vi "Apply (Greyscale Image).vi"(8 "error in (no error)":errorcluster, 9 "Destination Image in":T1, 10 "Greyscale Image in":T1, 11 "CLAHE in":refnum<class "CLAHE.lvclass">) -> (0 "error out":errorcluster, 2 "Destination Image":T1, 3 "CLAHE":refnum<class "CLAHE.lvclass">)   [LabVIEW 2020, in "image.lvlib" / "CLAHE.lvclass"]
uses:
  CLAHE.lvclass
  Greyscale Image.ctl
  CLAHE.lvclass/CLAHE.ctl
  common/common.lvlib
  common/bin/gartoolkit_32-1.dll
  image.lvlib
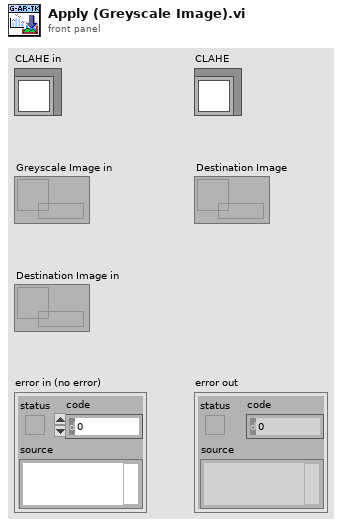
[diagram p1: front panel]
types:
  T1 = typedef "image.lvlib/Greyscale Image.ctl" = refnum<data-value>
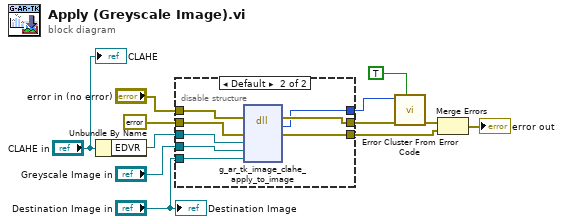
[diagram p0: block diagram]
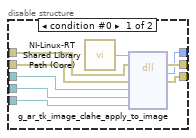
[diagram p2: hidden frame]
diagram:
  n1 = Unbundle By Name("CLAHE in") -> ("EDVR"=w1:refnum<data-value>)
  n2 = disable-structure shown="Default" {
    disable-tunnel: "error in (no error)" -> [w20 w29]
    disable-tunnel: errorcluster {"status"=FALSE, "code"=0, "source"=""} ("error constant") -> [w18 w28]
    disable-tunnel: w1 -> [w17 w24]
    disable-tunnel: [w19 w27] -> w10
    disable-tunnel: [w13 w26] -> w9
    disable-tunnel: [w14 w25] -> w8
    disable-tunnel: "Greyscale Image in" -> [w15 w23]
    disable-tunnel: "Destination Image in" -> [w16 w22]
    frame condition #0 {
      n3 = call "NI-Linux-RT Shared Library Path (Core).vi"() -> ("Path"=w21:path)
      n4 = dll-call lib="?" fn="g_ar_tk_image_clahe_apply_to_image" ("g_ar_toolkit.*.*:g_ar_tk_image_copy")(path in=w21, error in=w20, "error_cluster"=w18, "EDVR"=w17, "Source"=w15, "Destination"=w16) -> (error out=w19:errorcluster, "MgErrCode"=w13:i32, "error_cluster"=w14:errorcluster)  [unwired: 4 in, 1 out]
    }
    frame condition #1 (active) {
      n5 = dll-call lib="C:/serenial/lib/g-augmented-reality-toolkit/LabVIEW/common/bin/gartoolkit_*-1.*" fn="g_ar_tk_image_clahe_apply_to_image" ("g_ar_toolkit.*.*:g_ar_tk_image_copy")(error in=w29, "error_cluster"=w28, "EDVR"=w24, "Source"=w23, "Destination"=w22) -> (error out=w27:errorcluster, "MgErrCode"=w26:i32, "error_cluster"=w25:errorcluster)  [unwired: 5 in, 1 out]
    }
  }
  n6 = call <vilib>:"Error Cluster From Error Code.vi"("show call chain? (False)"=TRUE, "error in (no error)"=w10, "error code (0)"=w9) -> ("error out"=w12:errorcluster)  [unwired: 6 in]
  n7 = Merge Errors(w12, w8) -> (→"error out":errorcluster)
  "CLAHE" <- "CLAHE in"
  "Destination Image" <- "Destination Image in"
